vi "Prepare Data Modbus STS.vi"(10 "Direction":u16, 11 "Stand in":refnum<class "Stand.lvclass">) -> (3 "Data Write":T1)   [LabVIEW 2019, in "Stand.lvclass"]
uses:
  Stand.lvclass
  Modbus_class/WriteData.ctl
  Stand.lvclass/Stand.ctl
  AI_class/AI.lvclass/AI.ctl
  AnalogComparator_class/AnalogComparator.lvclass/AnalogComparator.ctl
  AnalogComparator_class/GetStatus.vi
  AI_class/AI.lvclass
  Modbus_class/ModbusSp.lvclass
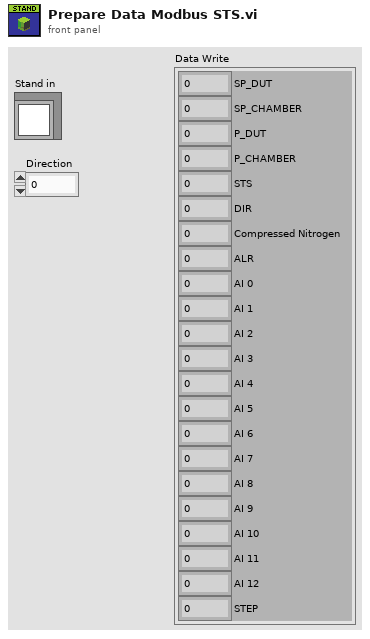
[diagram p1: front panel]
types:
  T1 = typedef "ModbusSp.lvclass/WriteData.ctl" = cluster{"SP_DUT":sgl, "SP_CHAMBER":sgl, "P_DUT":sgl, "P_CHAMBER":sgl, "STS":u16, "DIR":u16, "Compressed Nitrogen":u16, "ALR":u16, "AI 0":sgl, "AI 1":sgl, "AI 2":sgl, "AI 3":sgl, "AI 4":sgl, "AI 5":sgl, "AI 6":sgl, "AI 7":sgl, "AI 8":sgl, "AI 9":sgl, "AI 10":sgl, "AI 11":sgl, "AI 12":sgl, "STEP":u16}
  T2 = typedef "STS REG.ctl" = cluster{"IDLE":bool, "RYADY":bool, "STEP":bool, "ALARM":bool, "WARNING":bool, "REMOTE":bool, "SP_EXEC_DONE_DUT":bool, "SP_EXEC_DONE_CHAMBER":bool, "FILING_DONE_DUT":bool, "FILING_DONE_CHAMBER":bool, "BURETE_STATE":bool}
  T3 = typedef "Mode.ctl" = enum16{"IDLE", "FILLING", "EXECUTE_SP", "DRAIN"}
  T4 = typedef "AI_Data.ctl" = cluster{"Stat Data":T5, "OutOfRangeMax":bool, "OutOfRangeMin":bool, "HIHI":bool, "HI":bool, "LO":bool, "LOLO":bool}
  T5 = typedef "AI Statistics Data.ctl" = cluster{"raw mean":dbl, "scl mean":dbl, "raw mean 1Hz":dbl, "scl mean 1Hz":dbl}
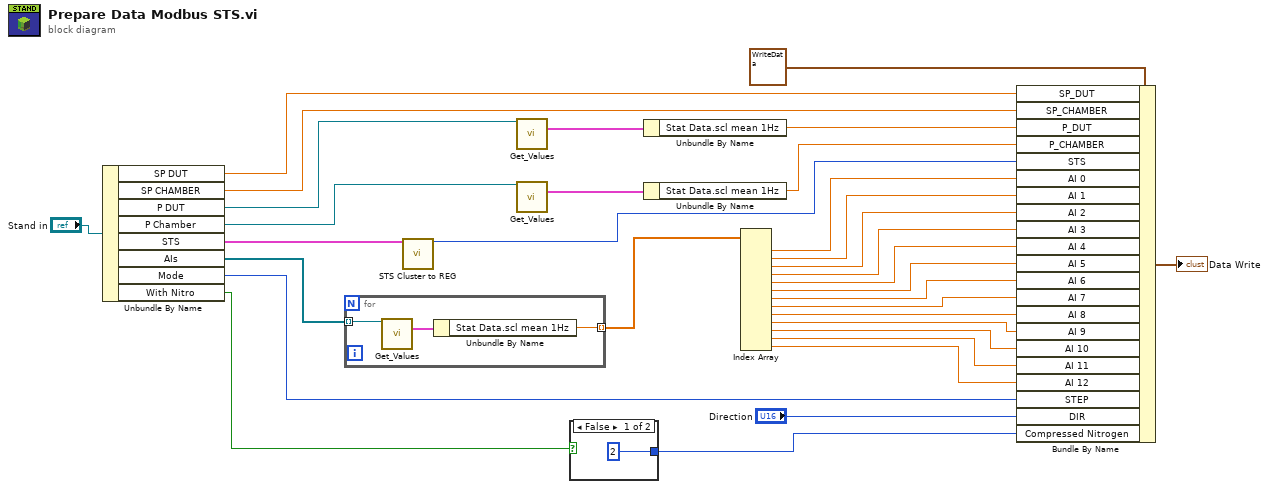
[diagram p0: block diagram]
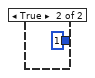
[diagram p2: hidden frame]
diagram:
  n1 = Unbundle By Name("Stand in") -> ("SP DUT"=w30:dbl, "SP CHAMBER"=w31:dbl, "P DUT"=w26:refnum<class "AI.lvclass">, "P Chamber"=w27:refnum<class "AI.lvclass">, "STS"=w7:T2, "AIs"=w28:refnum<class "AI.lvclass">[], "Mode"=w4:T3, "With Nitro"=w2:bool)
  n2 = for {
    tunnel: w28 -> [w35] mode=indexing
    tunnel: [w33] -> w9 mode=indexing
    n3 = call "Get_Values.vi"("reference in"=w35) -> ("Data"=w34:T4)  [unwired: 14 in]
    n4 = Unbundle By Name(w34) -> ("Stat Data.scl mean 1Hz"=w33:dbl)
  }
  n5 = call "STS Cluster to REG.vi"("STS REG"=w7) -> ("U16"=w21:u16)  [unwired: 14 in]
  n6 = call "Get_Values.vi"("reference in"=w26) -> ("Data"=w24:T4)  [unwired: 14 in]
  n7 = call "Get_Values.vi"("reference in"=w27) -> ("Data"=w25:T4)  [unwired: 14 in]
  n8 = case shown="False" w2 {
    tunnel: [u16 2 u16 1] -> w1
    frame False {
    }
    frame True {
    }
  }
  n9 = Unbundle By Name(w24) -> ("Stat Data.scl mean 1Hz"=w29:dbl)
  n10 = Unbundle By Name(w25) -> ("Stat Data.scl mean 1Hz"=w32:dbl)
  n11 = Index Array(array=w9) -> (element #1=w10:dbl, element #2=w11:dbl, element #3=w12:dbl, element #4=w13:dbl, element #5=w14:dbl, element #6=w15:dbl, element #7=w16:dbl, element #8=w17:dbl, element #9=w18:dbl, element #10=w19:dbl, element #11=w20:dbl, element #12=w6:dbl, element #13=w5:dbl)  [unwired: 13 in]
  n12 = Bundle By Name(cluster=T1 {"SP_DUT"=0.0, "SP_CHAMBER"=0.0, "P_DUT"=0.0, "P_CHAMBER"=0.0, "STS"=0, "DIR"=0, "Compressed Nitrogen"=0, "ALR"=0, "AI 0"=0.0, "AI 1"=0.0, "AI 2"=0.0, "AI 3"=0.0, "AI 4"=0.0, "AI 5"=0.0, "AI 6"=0.0, "AI 7"=0.0, "AI 8"=0.0, "AI 9"=0.0, "AI 10"=0.0, "AI 11"=0.0, "AI 12"=0.0, "STEP"=0} ("Data Write"), "SP_DUT"=w30, "SP_CHAMBER"=w31, "P_DUT"=w29, "P_CHAMBER"=w32, "STS"=w21, "AI 0"=w10, "AI 1"=w11, "AI 2"=w12, "AI 3"=w13, "AI 4"=w14, "AI 5"=w15, "AI 6"=w16, "AI 7"=w17, "AI 8"=w18, "AI 9"=w19, "AI 10"=w20, "AI 11"=w6, "AI 12"=w5, "STEP"=w4, "DIR"="Direction", "Compressed Nitrogen"=w1) -> (→"Data Write":T1)
